vi "emi_Numb S&E Messages in Q.vi"(11 "error in (no error)":errorcluster) -> (8 "# elements in queue":i32, 15 "error out":errorcluster)   [LabVIEW 2010]
doc: "Check teh number of S&E messages in the Q"
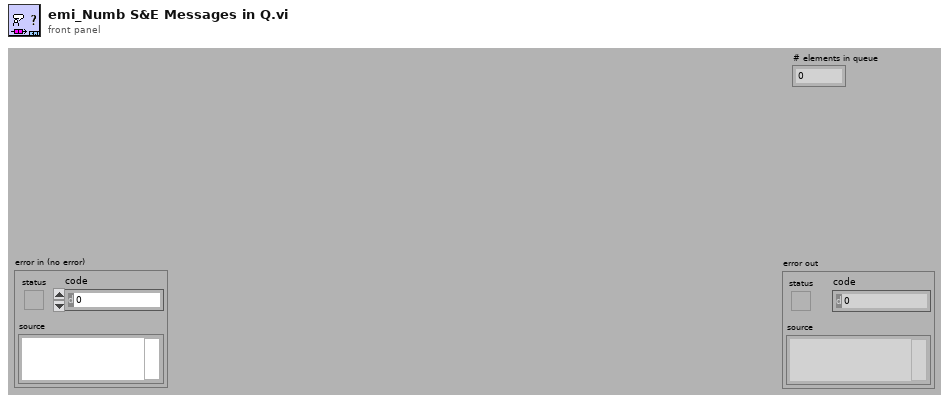
[diagram p1: front panel]
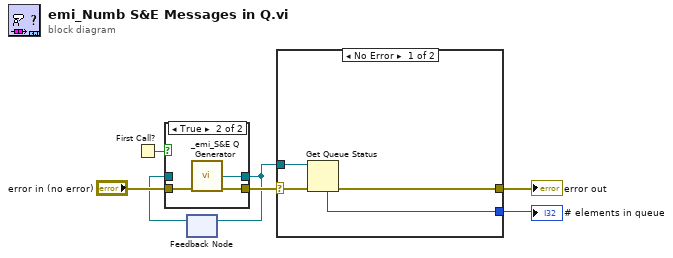
[diagram p0: block diagram]
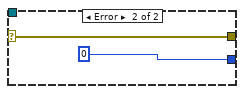
[diagram p3: hidden frame]
diagram:
  n1 = First Call?() -> (First Call?: T/F=w3:bool)
  n2 = feedback #1() -> (w4:refnum<queue>)  [unwired: 1 in]
  n3 = case shown="True" w3 {
    tunnel: "error in (no error)" -> [w8 w12]
    tunnel: [w8 w11] -> w5
    tunnel: [w9 w10] -> w2
    tunnel: w4 -> [w9 _]
    frame False {
    }
    frame True {
      n4 = call "_emi_S&E Q Generator.vi"("error in (no error)"=w12) -> ("E&S Message Q"=w10:refnum<queue>, "error out"=w11:errorcluster)  [unwired: 13 in]
    }
  }
  n5 = feedback-in #1(w2) -> ()
  n6 = case shown="No Error" w5 {
    selector: w5 -> [w16 w18]
    tunnel: [w15 w18] -> w7
    tunnel: w2 -> [w14 _]
    tunnel: [w13 0 ("# elements in queue")] -> w1
    frame No Error {
      n7 = Get Queue Status(queue=w14, error in (no error)=w16) -> (error out=w15:errorcluster, # elements in queue=w13:i32)  [unwired: 1 in, 6 out]
    }
    frame Error {
    }
  }
  "error out" <- w7
  "# elements in queue" <- w1
